vi "Get Node U16 Property.vi"(8 "Error In":errorcluster, 9 "Property Name":string, 10 "Node GUID":string, 11 "Root .NET Ref In":refnum<k24>) -> (0 "Error Out":errorcluster, 2 "Property":u16, 3 "Root .NET Ref Out":refnum<k24>)   [LabVIEW 2015]
doc: "Returns the specified U16 property of the first node found with the provided node GUID"
uses:
  NationalInstruments.VeriStand.SystemStorage
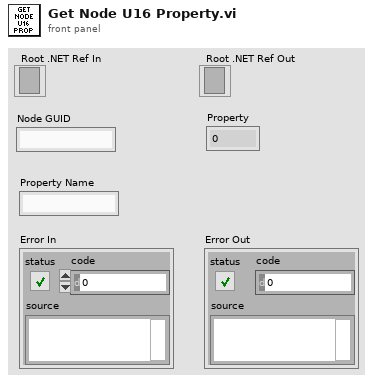
[diagram p1: front panel]
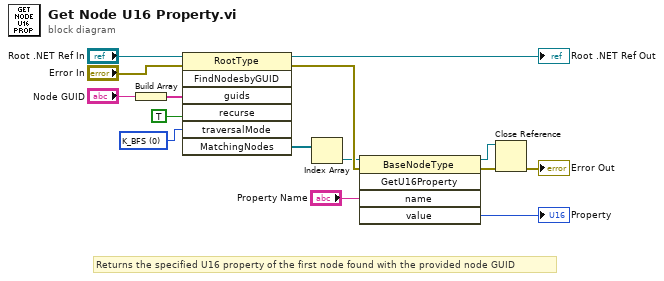
[diagram p0: block diagram]
diagram:
  w3 = 0 items=["K_BFS", "K_DFS", "K_CHILDONLY", "K_UP"] ("traversalMode")
  # "Returns the specified U16 property of the first node found with the provided node GUID"
  n1 = Build Array("Node GUID") -> (w1:string[])
  n2 = invoke class="RootType" method="FindNodesbyGUID"(reference="Root .NET Ref In", error in="Error In", "guids"=w1, "recurse"=TRUE, "traversalMode"=w3) -> (reference out=→"Root .NET Ref Out":refnum<k24>, error out=w10:errorcluster, "MatchingNodes"=w5:refnum<k24>[])  [unwired: 2 in, 4 out]
  n3 = Index Array(array=w5) -> (element=w9:refnum<k24>)  [unwired: 1 in]
  n4 = invoke class="BaseNodeType" method="GetU16Property"(reference=w9, error in=w10, "name"="Property Name") -> (reference out=w13:refnum<k24>, error out=w8:errorcluster, "value"=→"Property":u16)  [unwired: 2 in, 2 out]
  n5 = Close Reference(reference=w13, error in (no error)=w8) -> (error out=→"Error Out":errorcluster)
